vi "OAT Interpolation by Zero Insert (Real Input).vi"(7 "open interval?":bool=TRUE, 10 "L":i32, 11 "x":dbl[](array[numeric]) format="%.2f") -> (3 "y":dbl[](array[numeric]) format="%.2f")   [LabVIEW 2017, in "SoundVib_Resampling.lvlib"]
uses:
  <vilib>/addons/Sound and Vibration/Order Analysis/Resample Order Tracking/SoundVib_Resampling.lvlib
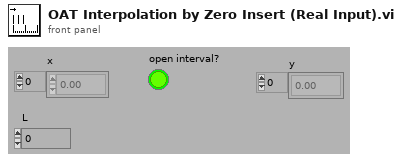
[diagram p1: front panel]
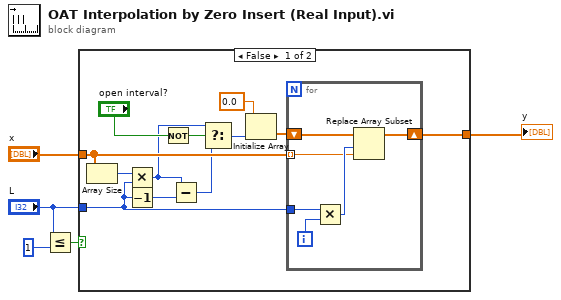
[diagram p0: block diagram]
diagram:
  n1 = Less Or Equal?(x="L", y=1) -> (x <= y?=w4:bool)
  n2 = case shown="False" w4 {
    tunnel: "x" -> [w15 w24]
    tunnel: "L" -> [w12 _]
    tunnel: [w13 w24] -> w1
    frame False {
      n3 = Array Size(array=w15) -> (size(s)=w14:i32)
      n4 = Multiply(x=w14, y=w12) -> (x*y=w6:i32)
      n5 = Decrement(x=w12) -> (x-1=w9:i32)
      n6 = Not(x="open interval?") -> (.not. x?=w8:bool)
      n7 = Subtract(x=w6, y=w9) -> (x-y=w7:i32)
      n8 = Select(t=w6, s=w8, f=w7) -> (s? t:f=w10:i32)
      n9 = Initialize Array(0.0 ("Element Data"), w10) -> (w16:dbl[])
      n10 = for {
        shift-right: [w21] -> w13
        shift-left: w16 -> [w22]
        tunnel: w15 -> [w18] mode=indexing
        tunnel: w12 -> [w19]
        i -> [w23]
        n11 = Multiply(x=w19, y=w23) -> (x*y=w20:i32)
        n12 = Replace Array Subset(array=w22, new element=w18, index=w20) -> (w21:dbl[])
      }
    }
    frame True {
    }
  }
  "y" <- w1
